vi "Null Broadcast Events--constant.vi"() -> (3 "Hardware Controller Broadcast Events":T1)   [LabVIEW 2024, in "Hardware Controller.lvlib"]
doc: "Returns the broadcast events cluster with null references for defining the event types in a Register For Events function.\n_____\nBased on DQMH Project Template 7.0.0.1280."
uses:
  Hardware Controller.lvlib
  Broadcast Events--cluster.ctl
  Did Init Argument--cluster.ctl
  Status Updated Argument--cluster.ctl
  Error Reported Argument--cluster.ctl
  Stop Argument--cluster.ctl
  Get Module Execution Status Argument--cluster.ctl
  System State Updated Argument--cluster.ctl
  EtherCAT Data Updated Argument--cluster.ctl
  System Fault Updated Argument--cluster.ctl
  EtherCAT Connection Status Updated Argument--cluster.ctl
  HardwareController IOLink Data Updated Argument--cluster.ctl
  IOLink Connection Updated Argument--cluster.ctl
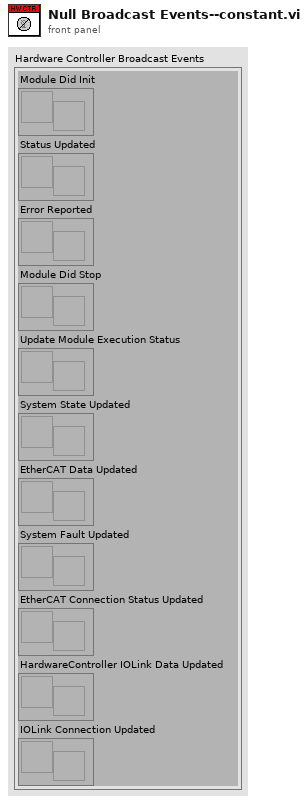
[diagram p1: front panel]
types:
  T1 = typedef "Hardware Controller.lvlib/Broadcast Events--cluster.ctl" = cluster{"Module Did Init":refnum<user-event>, "Status Updated":refnum<user-event>, "Error Reported":refnum<user-event>, "Module Did Stop":refnum<user-event>, "Update Module Execution Status":refnum<user-event>, "System State Updated":refnum<user-event>, "EtherCAT Data Updated":refnum<user-event>, "System Fault Updated":refnum<user-event>, "EtherCAT Connection Status Updated":refnum<user-event>, "HardwareController IOLink Data Updated":refnum<user-event>, "IOLink Connection Updated":refnum<user-event>}
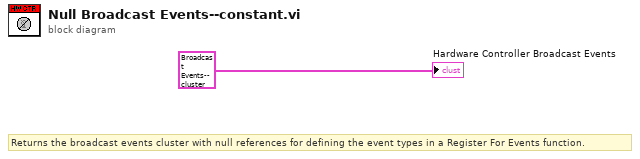
[diagram p0: block diagram]
diagram:
  # "Returns the broadcast events cluster with null references for defining the event types in a Register For Events function."
  "Hardware Controller Broadcast Events" <- T1 {"Module Did Init"=refnum, "Status Updated"=refnum, "Error Reported"=refnum, "Module Did Stop"=refnum, "Update Module Execution Status"=refnum, "System State Updated"=refnum, "EtherCAT Data Updated"=refnum, "System Fault Updated"=refnum, "EtherCAT Connection Status Updated"=refnum, "HardwareController IOLink Data Updated"=refnum, "IOLink Connection Updated"=refnum} ("Broadcast Events")
